vi "Construct Dialog Box Subscribes to Dbl X.vi"() -> (1 "Datum Received Notifier":refnum<notifier>, 3 "DialogBoxSubscribesToDblX":refnum<class "DialogBoxSubscribesToDblX.lvclass">)   [LabVIEW 2017, in "DialogBoxSubscribesToDblX.lvclass"]
uses:
  DialogBoxSubscribesToDblX.lvclass
  DialogBoxSubscribesToDblX.lvclass/DialogBoxSubscribesToDblX.ctl
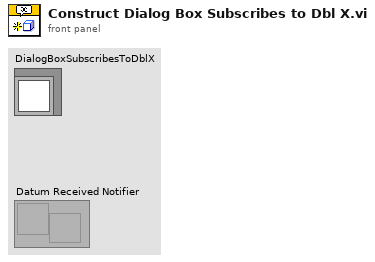
[diagram p1: front panel]
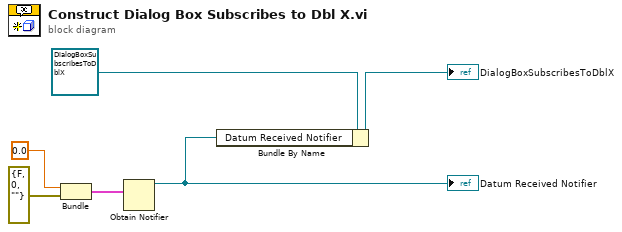
[diagram p0: block diagram]
diagram:
  n1 = Bundle(0.0, "error constant"=errorcluster {"status"=FALSE, "code"=0, "source"=""}) -> (w2:cluster{dbl, "error constant":errorcluster})  [unwired: 1 in]
  n2 = Obtain Notifier(notification data type=w2) -> (notifier out=w1:refnum<notifier>)  [unwired: 3 in, 2 out]
  "Datum Received Notifier" <- w1
  n3 = Bundle By Name(cluster=refnum<class "DialogBoxSubscribesToDblX.lvclass"> refnum ("DialogBoxSubscribesToDblX in"), "Datum Received Notifier"=w1) -> (→"DialogBoxSubscribesToDblX":refnum<class "DialogBoxSubscribesToDblX.lvclass">)
